vi "Front Panel2_ctrl.vi"() -> (0 "OK 2":bool)   [LabVIEW 2021]
uses:
  GL_SetpointDispl.vi
  GL_TempUnits.vi
  GL_SamplerateDispl.vi
  GL_Pgain.vi
  GL_Ireset.vi
  GL_Drate.vi
  GL_TempDspl.vi
  GL_MHeaterDisplay.vi
  GL_heaterdisplay.vi
  GL_HeaterOn.vi
panel:
  in  "ADJUST HEATER":bool
  out "Numeric 4":dbl format="%.2f"
  in  "Numeric 3":dbl format="%.2f"
  out "Numeric 2":dbl format="%.2f"
  in  "Numeric":i16
  in  "READ CALIBRATION":bool
  in  "SEND CALIBRATION":bool
  in  "D":dbl min=0.0 max=100.0 step=0.0001 format="%.2f"
  in  "I":dbl min=0.0 max=100.0 step=0.01 format="%.2f"
  in  "P":dbl min=0.0 max=100.0 step=0.01 format="%.2f"
  out "MANUAL HEATER DISPLAY":dbl(slide) caption="AMP" min=0.0 max=5.0 scale=0.0..5.0
  out "HEATER ON":bool
  out "Array":bool[](array[boolean])
  in  "SAMPLE RATE":dbl=1.0 min=0.0 max=600.0 step=0.001 format="%.3f"
  in  "SET POINT":dbl min=0.0 max=450.0 step=0.0001 format="%.3f"
  in  "unit":enum16{"K", "Ohms", "C", "F"}(ring)
  out "TEMPERATURE\nDisplay":dbl=1.0 min=1.0 max=450.0 format="%.3f"
  in  "OK":bool
  # "e"
  # "e"
  # "TEMPERATURE \nREMOTE TEMPERATURE CONTROLLER"
  # "TEMPERATURE \nREMOTE TEMPERATURE CONTROLLER"
  # "SET  POINT"
  # "SET  POINT"
  # "SAMPLE RATE"
  # "remote manual heater control\nnot functioning"
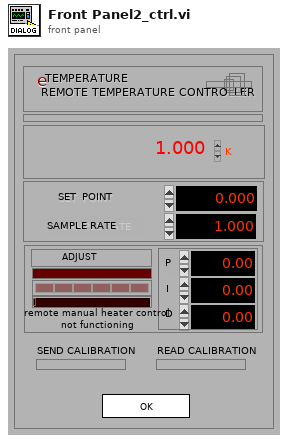
[diagram p1: front panel]
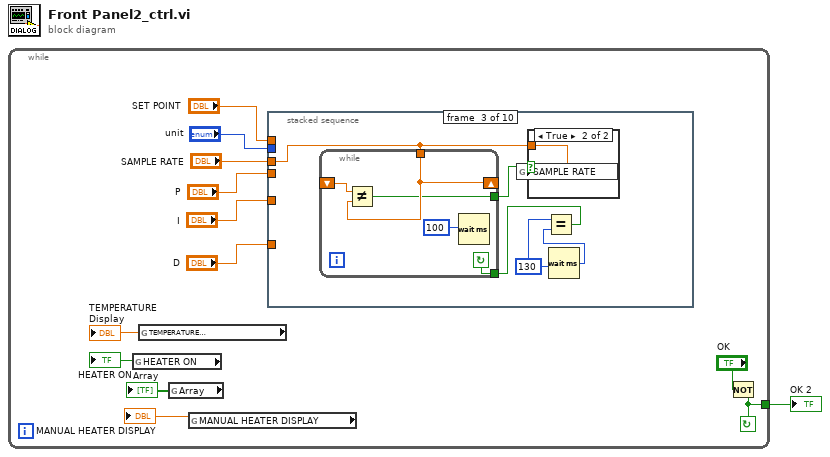
[diagram p0: block diagram]
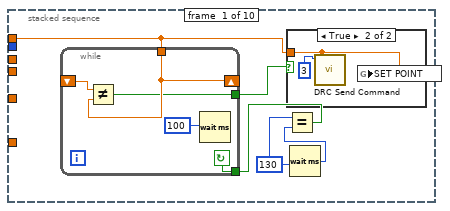
[diagram p2: hidden frame]
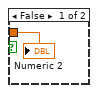
[diagram p3: hidden frame]
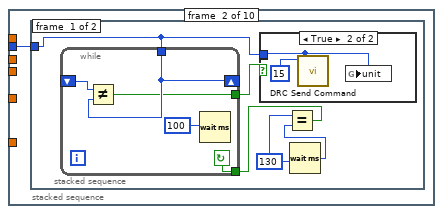
[diagram p4: hidden frame]
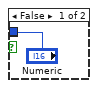
[diagram p5: hidden frame]
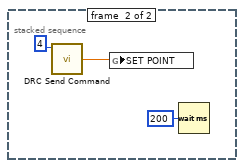
[diagram p6: hidden frame]
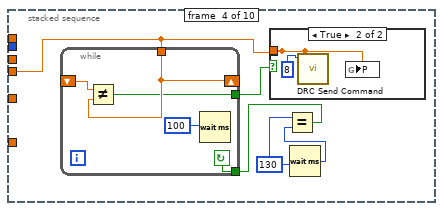
[diagram p8: hidden frame]
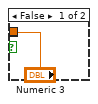
[diagram p9: hidden frame]
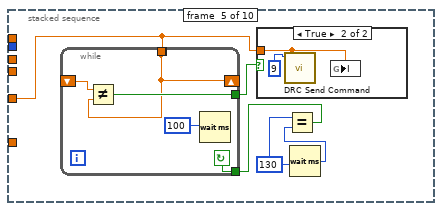
[diagram p10: hidden frame]
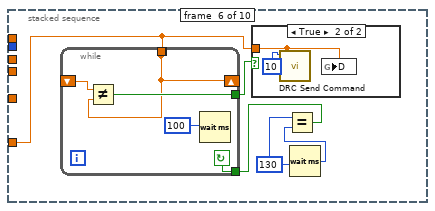
[diagram p12: hidden frame]
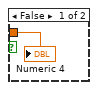
[diagram p13: hidden frame]
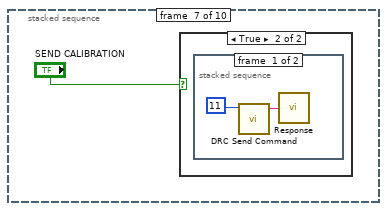
[diagram p14: hidden frame]
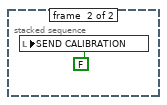
[diagram p16: hidden frame]
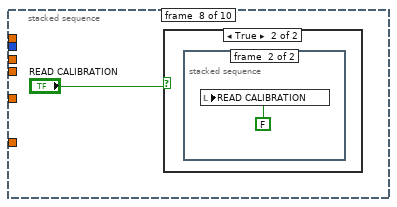
[diagram p17: hidden frame]
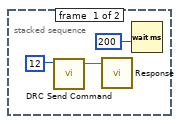
[diagram p19: hidden frame]
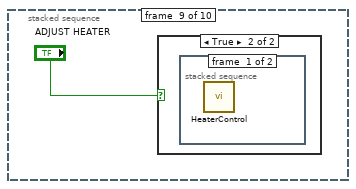
[diagram p20: hidden frame]
diagram:
  n1 = while {
    tunnel: [w12] -> w1
    stop <- w12 continue-if-true
    n2 = global read "GL_HeaterOn.vi" "HEATER ON"() -> (→"HEATER ON":bool)
    n3 = global read "GL_TempDspl.vi" "TEMPERATURE\nDisplay"() -> (→"TEMPERATURE\nDisplay":dbl)
    n4 = global read "GL_heaterdisplay.vi" "Array"() -> (→"Array":bool[])
    n5 = global read "GL_MHeaterDisplay.vi" "MANUAL HEATER DISPLAY"() -> (→"MANUAL HEATER DISPLAY":dbl)
    n6 = stacked-sequence {
      tunnel: "SET POINT" -> [w15 _ _ _ _ _ _ _ _ _]
      tunnel: "unit" -> [_ w27 _ _ _ _ _ _ _ _]
      tunnel: "SAMPLE RATE" -> [_ _ w44 _ _ _ _ _ _ w104]
      tunnel: "P" -> [_ _ _ w55 _ _ _ _ _ _]
      tunnel: "I" -> [_ _ _ _ w68 _ _ _ _ _]
      tunnel: "D" -> [_ _ _ _ _ w80 _ _ _ _]
      frame #0 {
        w18 = 130
        n7 = Wait (ms)(milliseconds to wait=w18) -> (millisecond timer value=w17:u32)
        n8 = Equal?(x=w18, y=w17) -> (x = y?=w16:bool)
        n9 = while {
          tunnel: w16 -> [w19]
          tunnel: [w20] -> w14
          tunnel: w15 -> [w21]
          shift-left: _ -> [w23]
          shift-right: [w21] -> _
          stop <- w19 continue-if-true
          n10 = Not Equal?(x=w23, y=w21) -> (x != y?=w20:bool)
          n11 = Wait (ms)(milliseconds to wait=100) -> ()  [unwired: 1 out]
        }
        n12 = case shown="True" w14 {
          tunnel: w15 -> [w24 w25]
          frame False {
            "Numeric 2" <- w24
          }
          frame True {
            n13 = call "DRC Send Command.vi"("Input"=w25, "Command"=3) -> ()  [unwired: 2 in, 3 out]
            n14 = global write "GL_SetpointDispl.vi" "SET POINT"(w25) -> ()
          }
        }
      }
      frame #1 {
        n15 = stacked-sequence {
          tunnel: w27 -> [w29 _]
          frame #0 {
            w32 = 130
            n16 = Wait (ms)(milliseconds to wait=w32) -> (millisecond timer value=w31:u32)
            n17 = Equal?(x=w32, y=w31) -> (x = y?=w30:bool)
            n18 = while {
              tunnel: w30 -> [w33]
              tunnel: [w34] -> w28
              tunnel: w29 -> [w35]
              shift-left: _ -> [w37]
              shift-right: [w35] -> _
              stop <- w33 continue-if-true
              n19 = Not Equal?(x=w37, y=w35) -> (x != y?=w34:bool)
              n20 = Wait (ms)(milliseconds to wait=100) -> ()  [unwired: 1 out]
            }
            n21 = case shown="True" w28 {
              tunnel: ["Numeric" w39] -> _
              tunnel: w29 -> [_ w39]
              frame False {
              }
              frame True {
                n22 = call "DRC Send Command.vi"("Input"=w39, "Command"=15) -> ()  [unwired: 2 in, 3 out]
                n23 = global write "GL_TempUnits.vi" "unit"(w39) -> ()
              }
            }
          }
          frame #1 {
            n24 = call "DRC Send Command.vi"("Command"=4) -> ("Output"=w42:dbl)  [unwired: 3 in, 2 out]
            n25 = global write "GL_SetpointDispl.vi" "SET POINT"(w42) -> ()
            n26 = Wait (ms)(milliseconds to wait=200) -> ()  [unwired: 1 out]
          }
        }
      }
      frame #2 {
        w48 = 130
        n27 = Wait (ms)(milliseconds to wait=w48) -> (millisecond timer value=w47:u32)
        n28 = Equal?(x=w48, y=w47) -> (x = y?=w46:bool)
        n29 = while {
          tunnel: w46 -> [w49]
          tunnel: [w50] -> w45
          tunnel: w44 -> [w51]
          shift-left: _ -> [w53]
          shift-right: [w51] -> _
          stop <- w49 continue-if-true
          n30 = Not Equal?(x=w53, y=w51) -> (x != y?=w50:bool)
          n31 = Wait (ms)(milliseconds to wait=100) -> ()  [unwired: 1 out]
        }
        n32 = case shown="True" w45 {
          tunnel: w44 -> [_ w54]
          frame False {
          }
          frame True {
            n33 = global write "GL_SamplerateDispl.vi" "SAMPLE RATE"(w54) -> ()
          }
        }
      }
      frame #3 {
        w59 = 130
        n34 = Wait (ms)(milliseconds to wait=w59) -> (millisecond timer value=w58:u32)
        n35 = Equal?(x=w59, y=w58) -> (x = y?=w57:bool)
        n36 = while {
          tunnel: [w60] -> w56
          tunnel: w57 -> [w61]
          tunnel: w55 -> [w62]
          shift-left: _ -> [w64]
          shift-right: [w62] -> _
          stop <- w61 continue-if-true
          n37 = Not Equal?(x=w64, y=w62) -> (x != y?=w60:bool)
          n38 = Wait (ms)(milliseconds to wait=100) -> ()  [unwired: 1 out]
        }
        n39 = case shown="True" w56 {
          tunnel: ["Numeric 3" w66] -> _
          tunnel: w55 -> [_ w66]
          frame False {
          }
          frame True {
            n40 = call "DRC Send Command.vi"("Input"=w66, "Command"=8) -> ()  [unwired: 2 in, 3 out]
            n41 = global write "GL_Pgain.vi" "P"(w66) -> ()
          }
        }
      }
      frame #4 {
        w72 = 130
        n42 = Wait (ms)(milliseconds to wait=w72) -> (millisecond timer value=w71:u32)
        n43 = Equal?(x=w72, y=w71) -> (x = y?=w70:bool)
        n44 = while {
          tunnel: w68 -> [w73]
          tunnel: w70 -> [w74]
          tunnel: [w75] -> w69
          tunnel: [w73] -> _
          shift-left: _ -> [w77]
          shift-right: [w73] -> _
          stop <- w74 continue-if-true
          n45 = Not Equal?(x=w77, y=w73) -> (x != y?=w75:bool)
          n46 = Wait (ms)(milliseconds to wait=100) -> ()  [unwired: 1 out]
        }
        n47 = case shown="True" w69 {
          tunnel: w68 -> [_ w78]
          frame False {
          }
          frame True {
            n48 = call "DRC Send Command.vi"("Input"=w78, "Command"=9) -> ()  [unwired: 2 in, 3 out]
            n49 = global write "GL_Ireset.vi" "I"(w78) -> ()
          }
        }
      }
      frame #5 {
        w84 = 130
        n50 = Wait (ms)(milliseconds to wait=w84) -> (millisecond timer value=w83:u32)
        n51 = Equal?(x=w84, y=w83) -> (x = y?=w82:bool)
        n52 = while {
          tunnel: w80 -> [w85]
          tunnel: w82 -> [w86]
          tunnel: [w87] -> w81
          tunnel: [w85] -> _
          shift-left: _ -> [w89]
          shift-right: [w85] -> _
          stop <- w86 continue-if-true
          n53 = Not Equal?(x=w89, y=w85) -> (x != y?=w87:bool)
          n54 = Wait (ms)(milliseconds to wait=100) -> ()  [unwired: 1 out]
        }
        n55 = case shown="True" w81 {
          tunnel: w80 -> [w90 w91]
          frame False {
            "Numeric 4" <- w90
          }
          frame True {
            n56 = call "DRC Send Command.vi"("Input"=w91, "Command"=10) -> ()  [unwired: 2 in, 3 out]
            n57 = global write "GL_Drate.vi" "D"(w91) -> ()
          }
        }
      }
      frame #6 {
        n58 = case shown="True" "SEND CALIBRATION" {
          frame False {
          }
          frame True {
            n59 = stacked-sequence {
              frame #0 {
                n60 = call "DRC Send Command.vi"("Command"=11) -> ("Response"=w94:string)  [unwired: 3 in, 2 out]
                n61 = call "Response.vi"("input String"=w94) -> ()  [unwired: 1 in, 2 out]
              }
              frame #1 {
                n62 = local write "SEND CALIBRATION"(FALSE) -> ()
              }
            }
          }
        }
      }
      frame #7 {
        n63 = case shown="True" "READ CALIBRATION" {
          frame False {
          }
          frame True {
            n64 = stacked-sequence {
              frame #0 {
                n65 = call "DRC Send Command.vi"("Command"=12) -> ("Response"=w98:string)  [unwired: 3 in, 2 out]
                n66 = call "Response.vi"("input String"=w98) -> ()  [unwired: 1 in, 2 out]
                n67 = Wait (ms)(milliseconds to wait=200) -> ()  [unwired: 1 out]
              }
              frame #1 {
                n68 = local write "READ CALIBRATION"(FALSE) -> ()
              }
            }
          }
        }
      }
      frame #8 {
        n69 = case shown="True" "ADJUST HEATER" {
          frame False {
          }
          frame True {
            n70 = stacked-sequence {
              frame #0 {
                n71 = call "HeaterControl.vi"() -> ()  [unwired: 4 in]
              }
              frame #1 {
                n72 = local write "ADJUST HEATER"(FALSE) -> ()
              }
            }
          }
        }
      }
      frame #9 {
        n73 = call "DRC Send Command.vi"("Command"=2) -> ("Output"=w105:dbl)  [unwired: 3 in, 2 out]
        n74 = global write "GL_TempDspl.vi" "TEMPERATURE\nDisplay"(w105) -> ()
        n75 = Multiply(x=w104, y=1000.0) -> (x*y=w107:dbl)
        n76 = Wait (ms)(milliseconds to wait=w107) -> ()  [unwired: 1 out]
      }
    }
    n77 = Not(x="OK") -> (.not. x?=w12:bool)
  }
  "OK 2" <- w1
